vi "Read Sender.vi"(8 "error in (no error)":errorcluster, 11 "Acquired Result in":refnum<class "Acquired Result.lvclass">) -> (0 "error out":errorcluster, 2 "Sender":string, 3 "Acquired Result out":refnum<class "Acquired Result.lvclass">)   [LabVIEW 2019, in "Acquired Result.lvclass"]
uses:
  Acquired Result.lvclass
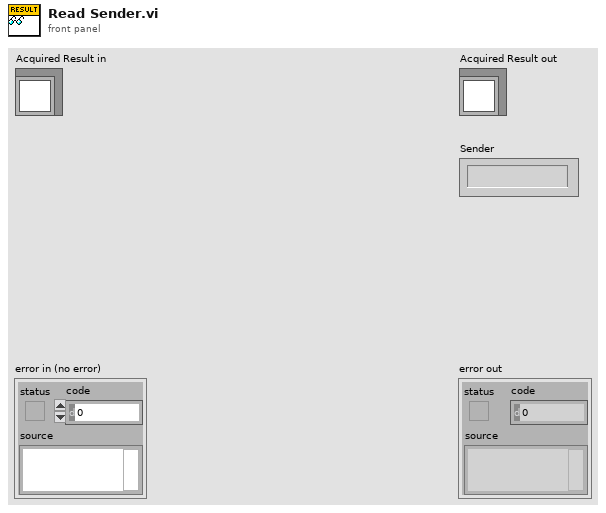
[diagram p1: front panel]
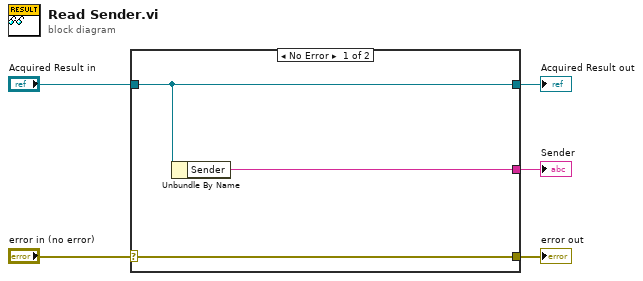
[diagram p0: block diagram]
diagram:
  n1 = case shown="No Error" "error in (no error)" {
    selector: "error in (no error)" -> [w8 w9]
    tunnel: [w8 w9] -> w4
    tunnel: [w7 w10] -> w2
    tunnel: "Acquired Result in" -> [w7 w10]
    tunnel: [w6 _] -> w1
    frame No Error {
      n2 = Unbundle By Name(w7) -> ("Sender"=w6:string)
    }
    frame Error {
    }
  }
  "error out" <- w4
  "Acquired Result out" <- w2
  "Sender" <- w1
